vi "Launch SW Actor.vi"(8 "error in (no error)":errorcluster, 11 "[MV] Key Certify in":refnum<class "[MV] Key Certify.lvclass">) -> (0 "error out":errorcluster, 3 "[MV] Key Certify out":refnum<class "[MV] Key Certify.lvclass">)   [LabVIEW 2020, in "[MV] Key Certify.lvlib" / "[MV] Key Certify.lvclass"]
uses:
  [MV] Key Certify.lvclass
  C:/Program Files/National Instruments/LabVIEW 2020/vi.lib/ActorFramework/Actor/Actor.lvclass
  <vilib>/ActorFramework/Actor/Actor.lvclass/Actor.ctl
  <vilib>/ActorFramework/Message Enqueuer/Message Enqueuer.lvclass/Message Enqueuer.ctl
  [MV] Key Certify.lvclass/[MV] Key Certify.ctl
  <vilib>/ActorFramework/Message Enqueuer/Init from Existing Queue.vi
  <vilib>/ActorFramework/Message Enqueuer/Enqueue.vi
  <vilib>/ActorFramework/Stop Msg/Stop Msg.lvclass
  C:/Program Files/National Instruments/LabVIEW 2020/vi.lib/ActorFramework/Message/Message.lvclass
  <vilib>/ActorFramework/Message Priority Queue/Priority Enqueue.vi
  <vilib>/ActorFramework/Message Enqueuer/Message Enqueuer.lvclass
  <vilib>/ActorFramework/Actor/Actor.lvclass
  D:/2_GitHub/LabVIEW-Key/Key Certify/[MV] Key Certify/[MV] Key Certify/[MV] Key Certify.lvclass
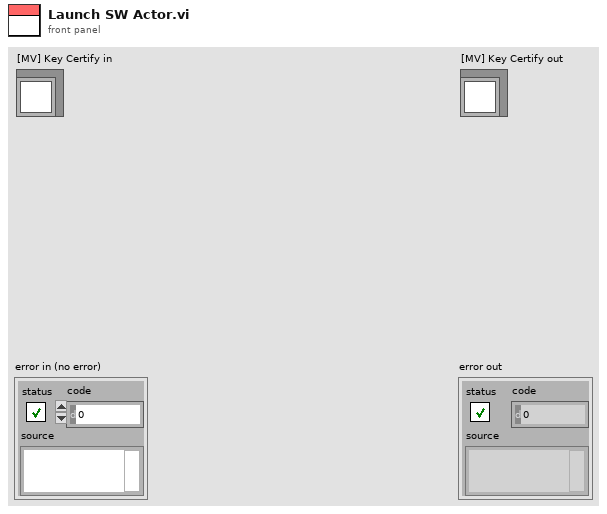
[diagram p1: front panel]
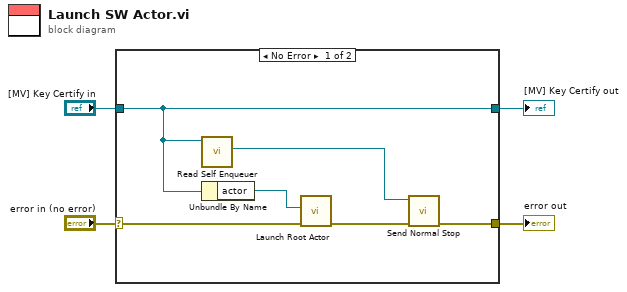
[diagram p0: block diagram]
diagram:
  n1 = case shown="No Error" "error in (no error)" {
    selector: "error in (no error)" -> [w10 w12]
    tunnel: [w8 w12] -> w3
    tunnel: [w9 w11] -> w1
    tunnel: "[MV] Key Certify in" -> [w9 w11]
    frame No Error {
      n2 = call <vilib>:"Read Self Enqueuer.vi"("Actor"=w9) -> ("Self Enqueuer"=w7:refnum<class "Message Enqueuer.lvclass">)  [unwired: 10 in]
      n3 = Unbundle By Name(w9) -> ("actor"=w6:refnum<class "Actor.lvclass">)
      n4 = call <vilib>:"Launch Root Actor.vi"("error in (no error)"=w10, "Actor"=w6) -> ("error out"=w5:errorcluster)  [unwired: 8 in, 1 out]
      n5 = call <vilib>:"Send Normal Stop.vi"("error in (no error)"=w5, "Message Enqueuer"=w7) -> ("error out"=w8:errorcluster)  [unwired: 9 in]
    }
    frame Error {
    }
  }
  "error out" <- w3
  "[MV] Key Certify out" <- w1
